vi "DrawGraphics.vi"() -> ()   [LabVIEW 2017]
panel:
  in  "Tab Control":enum32{"Circle", "Line"}(tab)
  in  "Radius":dbl
  in  "Origin":cluster{"x":dbl, "y":dbl}
  in  "End":cluster{"x":dbl, "y":dbl}
  in  "Start":cluster{"x":dbl, "y":dbl}
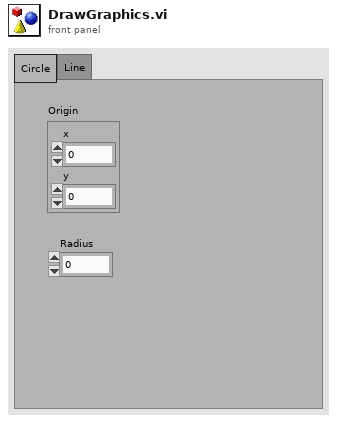
[diagram p1: front panel]
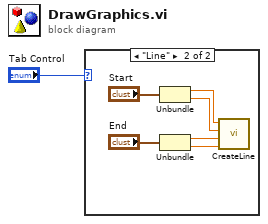
[diagram p0: block diagram]
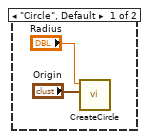
[diagram p2: hidden frame]
diagram:
  n1 = case shown="\"Line\"" "Tab Control" {
    frame "Circle", Default {
      n2 = call "CreateCircle.vi"("Origin"="Origin", "Radius"="Radius") -> ()  [unwired: 10 in]
    }
    frame "Line" {
      n3 = Unbundle("Start") -> ("x"=w8:dbl, "y"=w7:dbl)
      n4 = Unbundle("End") -> ("x"=w5:dbl, "y"=w4:dbl)
      n5 = call "CreateLine.vi"("endY"=w4, "endX"=w5, "startY"=w7, "startX"=w8) -> ()  [unwired: 8 in]
    }
  }
